vi "Simplify_Mult_Assign.vi"(11 "Parse Tree in":T1[](array[typedef])=[{"parent"=0, "children"=[1], "token"="[STAT_LST]", "NodeType"=enum."statement_list", "line"=0, "display"=FALSE, "position"=0, "uniqueid"=0}, {"parent"=0, "children"=[2, 4, 5], "token"="=", "NodeType"=enum."assignment", "line"=1, "display"=FALSE, "position"=10, "uniqueid"=1}, {"parent"=1, "children"=[3], "token"="a", "NodeType"=enum."identifier", "line"=1, "display"=FALSE, "position"=2, "uniqueid"=2}, {"parent"=2, "children"=[], "token"="1", "NodeType"=enum."constant", "line"=1, "display"=FALSE, "position"=4, "uniqueid"=3}, {"parent"=1, "children"=[], "token"="b", "NodeType"=enum."identifier", "line"=1, "display"=FALSE, "position"=7, "uniqueid"=4}, {"parent"=1, "children"=[6], "token"="max", "NodeType"=enum."function_1_N", "line"=1, "display"=FALSE, "position"=12, "uniqueid"=5}, {"parent"=5, "children"=[], "token"="x", "NodeType"=enum."function_0_1", "line"=1, "display"=FALSE, "position"=16, "uniqueid"=6}]) -> (3 "Parse Tree":T1[](array[typedef]))   [LabVIEW 2021]
uses:
  <resource>/MathScriptParser/Statement.ctl
  <resource>/MathScriptParser/NodeType.ctl
  <vilib>/imath/engines/lvmath2/StdLib/Stack/Stack(I32).llb/Stack(I32).lvclass
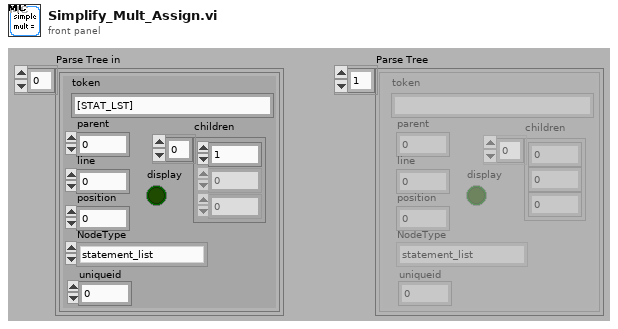
[diagram p1: front panel]
types:
  T1 = typedef "Statement.ctl" = cluster{"parent":u32, "children":u32[], "token":string, "NodeType":T2, "line":u32, "display":bool, "position":u32, "uniqueid":u32}
  T2 = typedef "NodeType.ctl" = enum16{"statement_list", "expression_list", "matrix", "row", "command", "function_1_1", "function_1_N", "function_N_1", "function_N_N", "operator", "assignment", "for", "if", "switch", "while", "try", "range", "identifier", "struct_field", "constant", "udfunction_1_1", "udfunction_1_N", "udfunction_N_1", "udfunction_N_N", "udfunction_0_0", "udfunction_0_1", "udfunction_0_N", "udfunction_1_0", "udfunction_N_0", "function_0_1", "function_0_N", "struct_ref", "array_ref", "cell_array_ref", "cell_matrix"}
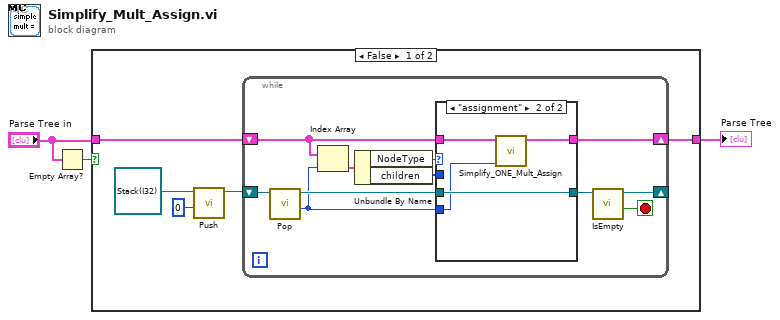
[diagram p0: block diagram]
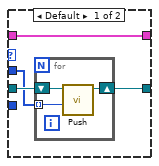
[diagram p2: hidden frame]
diagram:
  n1 = Empty Array?(array="Parse Tree in") -> (empty?=w2:bool)
  n2 = case shown="False" w2 {
    tunnel: "Parse Tree in" -> [w5 w31]
    tunnel: [w4 w31] -> w3
    frame False {
      n3 = call <vilib>:"Push.vi"("Element"=0, "Stack(I32) in"=refnum<class "Stack(I32).lvclass"> refnum ("Stack(I32).lvclass")) -> ("Stack(I32) out"=w6:refnum<class "Stack(I32).lvclass">)  [unwired: 9 out]
      n4 = while {
        shift-right: [w9] -> _
        shift-left: w6 -> [w18]
        shift-right: [w11] -> w4
        shift-left: w5 -> [w12]
        stop <- w19 stop-if-true
        n5 = call <vilib>:"Pop.vi"("Stack(I32) in"=w18) -> ("Element"=w13:i32, "Stack(I32) out"=w14:refnum<class "Stack(I32).lvclass">)  [unwired: 9 out]
        n6 = Index Array(array=w12, index=w13) -> (element=w17:T1)
        n7 = Unbundle By Name(w17) -> ("NodeType"=w16:T2, "children"=w15:u32[])
        n8 = case shown="\"assignment\"" w16 {
          tunnel: w15 -> [w21 _]
          tunnel: w14 -> [w23 w30]
          tunnel: [w22 w30] -> w10
          tunnel: w13 -> [_ w27]
          tunnel: w12 -> [w20 w29]
          tunnel: [w20 w28] -> w11
          frame Default {
            n9 = for {
              shift-right: [w25] -> w22
              shift-left: w23 -> [w26]
              tunnel: w21 -> [w24] mode=indexing
              n10 = call <vilib>:"Push.vi"("Element"=w24, "Stack(I32) in"=w26) -> ("Stack(I32) out"=w25:refnum<class "Stack(I32).lvclass">)  [unwired: 9 out]
            }
          }
          frame "assignment" {
            n11 = call <vilib>:"Simplify_ONE_Mult_Assign.vi"("Assignment Statement"=w27, "Parse Tree in"=w29) -> ("Parse Tree"=w28:T1[])  [unwired: 9 out]
          }
        }
        n12 = call <vilib>:"IsEmpty.vi"("Stack(I32) in"=w10) -> ("IsEmpty?"=w19:bool, "Stack(I32) out"=w9:refnum<class "Stack(I32).lvclass">)  [unwired: 9 out]
      }
    }
    frame True {
    }
  }
  "Parse Tree" <- w3
